vi "Destroy User Event.vi"(8 "error in (no error)":errorcluster caption="에러 입력(에러 없음)", 11 "User Event":refnum<user-event>) -> (0 "error out":errorcluster caption="에러 출력")   [LabVIEW 2018, in "User Event.lvlib"]
uses:
  User Event.lvlib
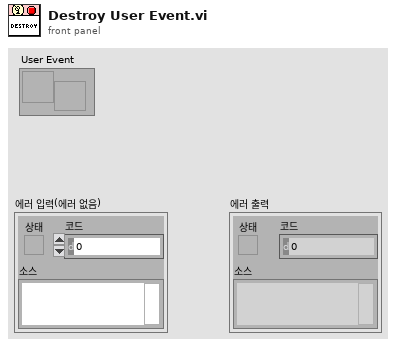
[diagram p1: front panel]
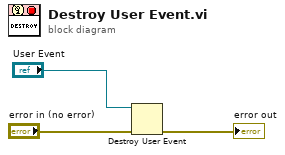
[diagram p0: block diagram]
diagram:
  n1 = Destroy User Event(user event="User Event", error in="error in (no error)") -> (error out=→"error out":errorcluster)
